vi "Calling VI in Class B.vi"   [LabVIEW 2023, in "Class B.lvclass"]
doc: "This VI is a member of Class B."
uses:
  Class B.lvclass
  Class A/Class A.lvclass
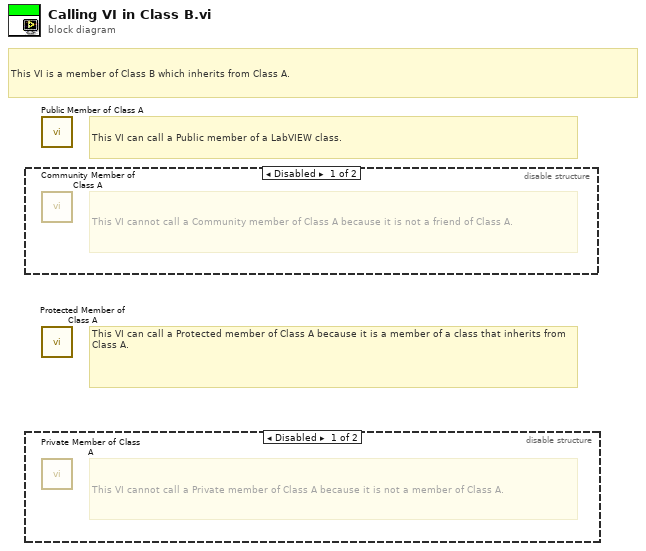
[diagram p0: block diagram]
diagram:
  # "This VI can call a Protected member of Class A because it is a member of a class that inherits from Class A."
  # "This VI can call a Public member of a LabVIEW class."
  # "This VI is a member of Class B which inherits from Class A."
  n1 = disable-structure shown="Disabled" {
    frame Disabled {
      # "This VI cannot call a Community member of Class A because it is not a friend of Class A."
      n2 = call "Community Member of Class A.vi"() -> ()  [unwired: 12 in]
    }
    frame Enabled {
    }
  }
  n3 = disable-structure shown="Disabled" {
    frame Disabled {
      # "This VI cannot call a Private member of Class A because it is not a member of Class A."
      n4 = call "Private Member of Class A.vi"() -> ()  [unwired: 12 in]
    }
    frame Enabled {
    }
  }
  n5 = call "Public Member of Class A.vi"() -> ()  [unwired: 12 in]
  n6 = call "Protected Member of Class A.vi"() -> ()  [unwired: 12 in]
